vi "contadorcajas.vi"() -> ()   [LabVIEW 2020]
uses:
  <vilib>/MakerHub/LINX/Public/Peripherals/Digital/Digital Read 1 Chan.vi
  <vilib>/MakerHub/LINX/Public/Peripherals/Digital/Digital Read N Chans.vi
  <vilib>/MakerHub/LINX/Private/Local IO/LinxDigitalRead.vi
  <vilib>/MakerHub/LINX/Public/Utilities/Check Channel.vi
  <vilib>/MakerHub/LINX/Public/Utilities/Open Serial.vi
  <vilib>/MakerHub/LINX/Private/Utilties/Generate Error.vi
  <vilib>/MakerHub/LINX/LMH-LINX.lvlib
  <vilib>/ptbypt/NI_PtbyPt.lvlib
panel:
  in  "Reset":bool
  in  "tamaño de lineas en mm":dbl
  in  "DI Channel  detector":u8
  in  "DI Channel pulso":u8
  in  "Serial Port":refnum<visa-resource-name>
  out "Medidas de caja en mm":dbl
  out "Pulso":bool
  out "Detector":bool
  out "CONTADOR":dbl
  in  "?":bool
  # "LINX AJUSTES DEL DISPOSITIVO"
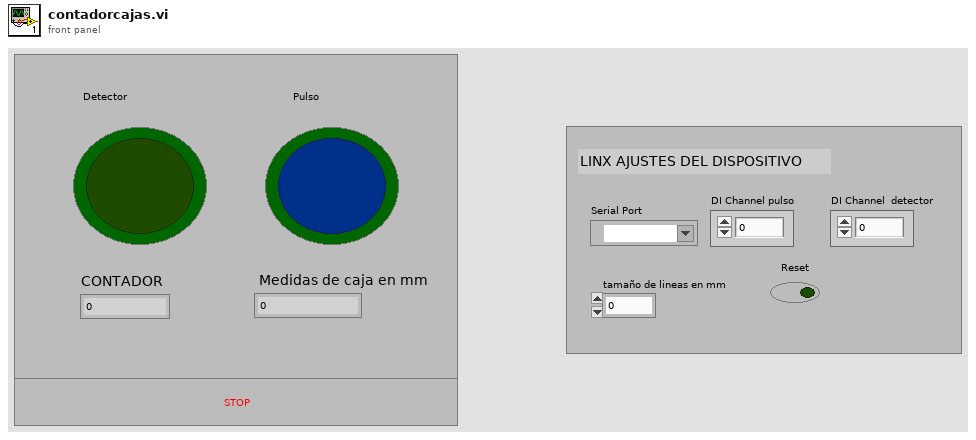
[diagram p1: front panel]
types:
  T1 = typedef "LMH-LINX.lvlib/LINX Ref.ctl" = cluster{"IO":T2, "Interface":T3, "LINX Device Config":T4}
  T2 = typedef "LMH-LINX.lvlib/Platform.ctl" = enum16{"Remote", "Local"}
  T3 = typedef "LMH-LINX.lvlib/Interface.ctl" = enum16{"Serial", "TCP"}
  T4 = typedef "LMH-LINX.lvlib/Device.lvlib/LINX Device Config.ctl" = cluster{"Interface":T3, "COM Port":refnum<visa-resource-name>, "TCP Configuration":T5, "Device Family":u8, "Device ID":u8, "Device Name":string, "TCP Ref":refnum<k5>, "Channels":T6}
  T5 = typedef "LMH-LINX.lvlib/Device.lvlib/TCP Config.ctl" = cluster{"IP Address":string, "Port":u16}
  T6 = typedef "LMH-LINX.lvlib/Channels.ctl" = cluster{"DI":u8[], "DO":u8[], "AI":u8[], "AO":u8[], "PWM":u8[], "QE":u8[], "UART":u8[], "I2C 2":u8[], "SPI":u8[], "CAN":u8[], "Servo":u8[], "AI Ref (V)":dbl, "AI Resolution (Bits)":u8, "AO Ref (V)":dbl, "AO Resolution (Bits)":u8}
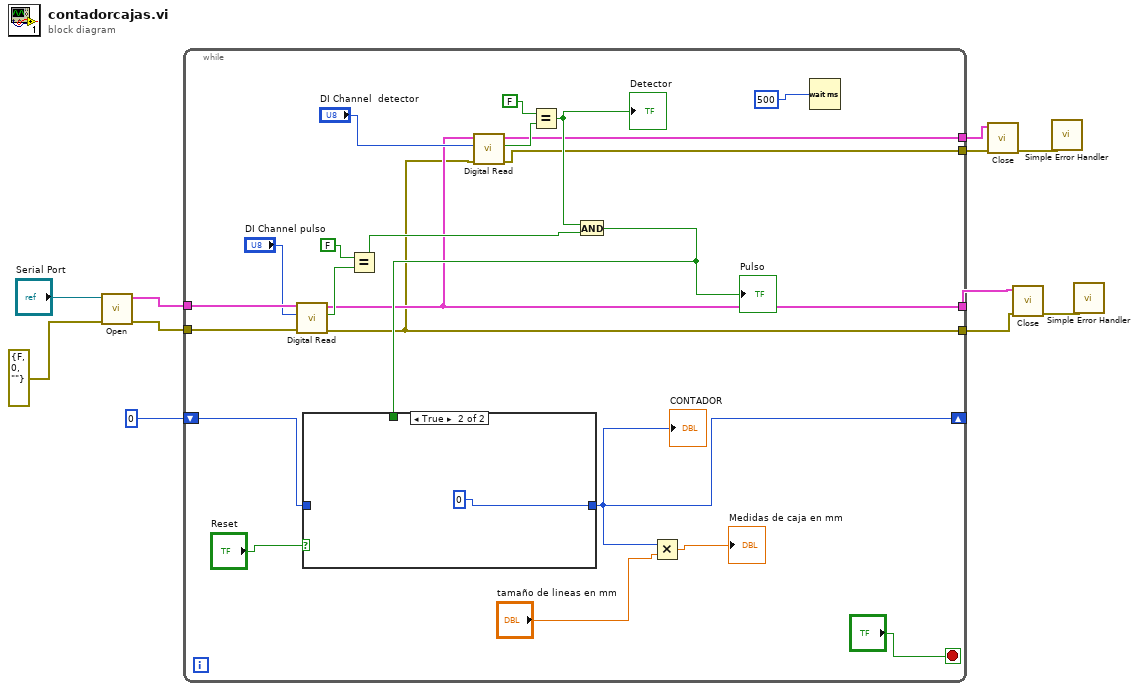
[diagram p0: block diagram]
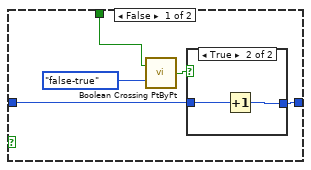
[diagram p2: hidden frame]
diagram:
  n1 = call-poly <vilib>:"Open.vi"("Error In"=errorcluster {"status"=FALSE, "code"=0, "source"=""} ("error constant"), "Serial Port"="Serial Port") -> ("Error Out"=w8:errorcluster, "LINX Resource"=w9:T1)  [unwired: 7 in, 1 out]
  n2 = while {
    tunnel: w9 -> [w33]
    tunnel: w8 -> [w32]
    shift-right: [w17] -> _
    shift-left: 0 -> [w22]
    tunnel: [w16] -> w6
    tunnel: [w15] -> w5
    tunnel: [w14] -> w3
    tunnel: [w13] -> w2
    stop <- "?" stop-if-true
    n3 = call-poly <vilib>:"Digital Read.vi"("Error In"=w32, "DI Channel"="DI Channel pulso", "LINX Resource"=w33) -> ("Error Out"=w13:errorcluster, "DI Value"=w30:bool, "LINX Resource"=w14:T1)  [unwired: 6 in]
    n4 = Equal?(x=FALSE, y=w30) -> (x = y?=w24:bool)
    n5 = call-poly <vilib>:"Digital Read.vi"("Error In"=w13, "DI Channel"="DI Channel  detector", "LINX Resource"=w14) -> ("Error Out"=w15:errorcluster, "DI Value"=w26:bool, "LINX Resource"=w16:T1)  [unwired: 6 in]
    n6 = Equal?(x=FALSE, y=w26) -> (x = y?=w25:bool)
    "Detector" <- w25
    n7 = And(x=w25, y=w24) -> (x .and. y?=w23:bool)
    "Pulso" <- w23
    n8 = case shown="True" "Reset" {
      tunnel: [w38 0] -> w17
      tunnel: w22 -> [w37 _]
      tunnel: w23 -> [w35 _]
      frame False {
        n9 = call <vilib>:"Boolean Crossing PtByPt.vi"("direction"=enum16{"either", "false-true", "true-false"}."false-true", "input"=w35) -> ("crossing"=w36:bool)  [unwired: 1 in]
        n10 = case shown="True" w36 {
          tunnel: [w39 w41] -> w38
          tunnel: w37 -> [w39 w40]
          frame False {
          }
          frame True {
            n11 = Increment(x=w40) -> (x+1=w41:i32)
          }
        }
      }
      frame True {
      }
    }
    "CONTADOR" <- w17
    n12 = Multiply(x=w17, y="tamaño de lineas en mm") -> (x*y=→"Medidas de caja en mm":dbl)
    n13 = Wait (ms)(milliseconds to wait=500) -> ()  [unwired: 1 out]
  }
  n14 = call <vilib>:"Close.vi"("Error In"=w5, "LINX Resource"=w6) -> ("Error Out"=w4:errorcluster)  [unwired: 9 in]
  n15 = call <vilib>:"Close.vi"("Error In"=w2, "LINX Resource"=w3) -> ("Error Out"=w1:errorcluster)  [unwired: 9 in]
  n16 = call <vilib>:"Simple Error Handler.vi"("error in (no error)"=w4) -> ()  [unwired: 4 in, 5 out]
  n17 = call <vilib>:"Simple Error Handler.vi"("error in (no error)"=w1) -> ()  [unwired: 4 in, 5 out]
